vi "Sim GPS.vi"() -> ()   [LabVIEW 2012]
uses:
  <instrlib>/Garmin GPS Series/HAIOL/Simulator/Garmin GPS Series Simulator.lvclass
  <instrlib>/Garmin GPS Series/HAIOL/Garmin GPS Series.lvclass
  <vilib>/Platform/TimedLoop/XDataNode/XDataNode.xnode
  <vilib>/Platform/TimedLoop/XDataNode/nitl_modes.ctl
  <vilib>/Platform/TimedLoop/XDataNode/XDNodeRunTimeDep.lvlib
  <vilib>/Platform/TimedLoop/XDataNode/wakeup.ctl
  <vilib>/Platform/TimedLoop/XDataNode/timing_clust.ctl
panel:
  in  "error in (no error)":errorcluster
  in  "stop?":bool
  out "GPS Data":T1 {"Time"."GPS Time of Week" format="%.3f"; "Velocity, Correction & SET"."Extended Navigation Mode" items=["Non Differential"=0, "Code (RTCM Type 1 & 9)"=1, "Code, Single Frequency (WAAS)"=2, "Code, Dual Frequency (WAAS)"=3, "Code, Single Frequency (WCT)"=4, "Code/RCP, Dual Frequency (WCT)"=5, "Code, Single Frequency (RTG)"=6, "Code (RTCM Type 1 & 9) Dual Frequency"=10, "Code/RCP, Dual Frequency (RTG)"=11, "Code, Single Frequency (NCT-RTK)"=12, "Code, Single Frequency (RTCM 18 & 19)"=13, "Code, Single Frequency (RTCM 21 & 22)"=14, "Code, Single Frequency (CMR)"=15, "Code, Dual Frequency (NCT-RTK)"=16, "Code, Dual Frequency (RTCM 18 & 19)"=17, "Code, Dual Frequency (RTCM 20 & 21)"=18, "Code, Dual Frequency (CMR)"=19, "RTK (NCT-RTK)"=20, "RTK (RTCM 18 & 19)"=21, "RTK (RTCM 20 & 21)"=22, "RTK (CMR)"=23, "Code, Single Frequency with SET (RTG)"=24, "Code/RCP, Dual Frequency with SET (RTG)"=25, "RTK Extend"=26]; "Altitude" format="%#_18g"; "Longitude" format="%#_18g"; "Latitude" format="%#_18g"}
  in  "GPS Data Cluster":T1 {"Time"."GPS Time of Week" format="%.3f"; "Velocity, Correction & SET"."Extended Navigation Mode" items=["Non Differential"=0, "Code (RTCM Type 1 & 9)"=1, "Code, Single Frequency (WAAS)"=2, "Code, Dual Frequency (WAAS)"=3, "Code, Single Frequency (WCT)"=4, "Code/RCP, Dual Frequency (WCT)"=5, "Code, Single Frequency (RTG)"=6, "Code (RTCM Type 1 & 9) Dual Frequency"=10, "Code/RCP, Dual Frequency (RTG)"=11, "Code, Single Frequency (NCT-RTK)"=12, "Code, Single Frequency (RTCM 18 & 19)"=13, "Code, Single Frequency (RTCM 21 & 22)"=14, "Code, Single Frequency (CMR)"=15, "Code, Dual Frequency (NCT-RTK)"=16, "Code, Dual Frequency (RTCM 18 & 19)"=17, "Code, Dual Frequency (RTCM 20 & 21)"=18, "Code, Dual Frequency (CMR)"=19, "RTK (NCT-RTK)"=20, "RTK (RTCM 18 & 19)"=21, "RTK (RTCM 20 & 21)"=22, "RTK (CMR)"=23, "Code, Single Frequency with SET (RTG)"=24, "Code/RCP, Dual Frequency with SET (RTG)"=25, "RTK Extend"=26]}
  out "error out":errorcluster
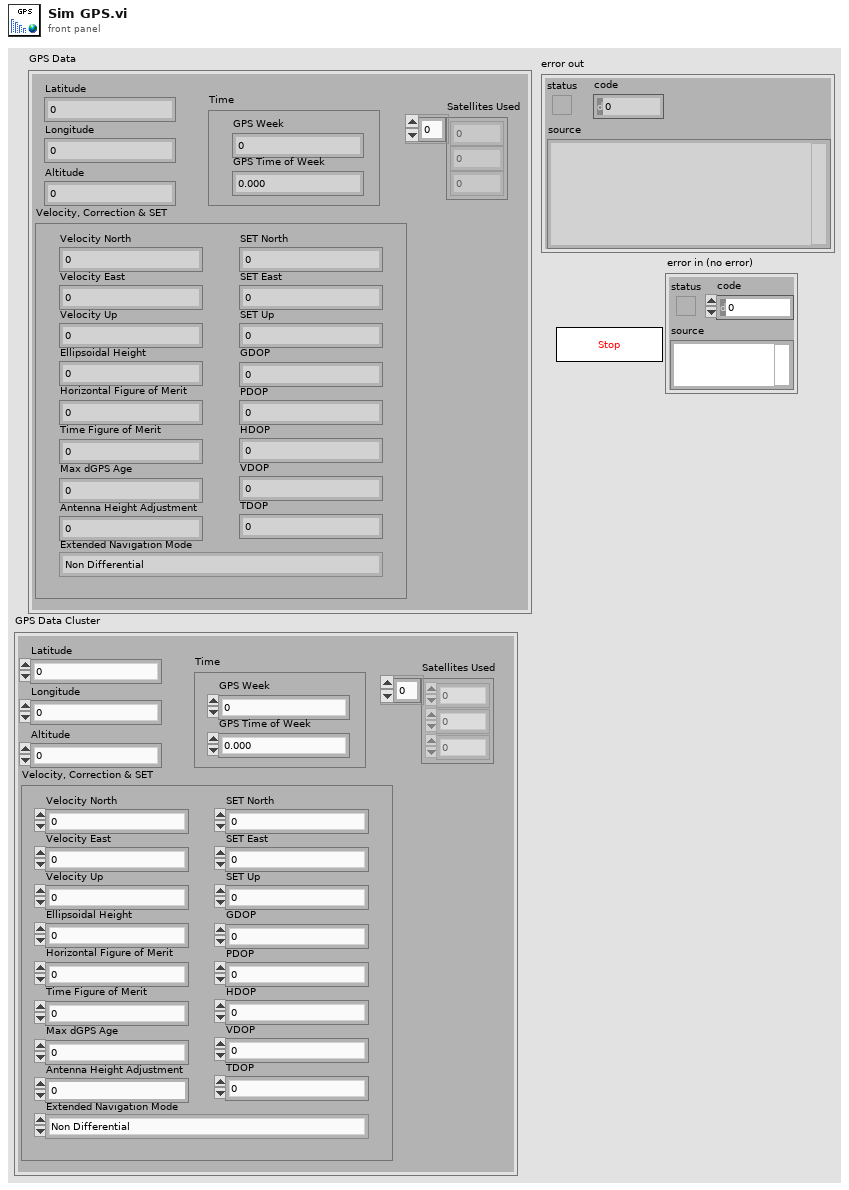
[diagram p1: front panel]
types:
  T1 = cluster{"Latitude":dbl, "Longitude":dbl, "Altitude":dbl, "Velocity, Correction & SET":cluster{"Velocity North":dbl, "Velocity East":dbl, "Velocity Up":dbl, "Ellipsoidal Height":dbl, "GDOP":sgl, "PDOP":sgl, "HDOP":sgl, "VDOP":sgl, "TDOP":sgl, "Horizontal Figure of Merit":u8, "Time Figure of Merit":u8, "Max dGPS Age":sgl, "Extended Navigation Mode":u8, "Antenna Height Adjustment ":dbl, "SET North":i32, "SET East":i32, "SET Up":i32}, "Time":cluster{"GPS Week":u16, "GPS Time of Week":sgl}, "Satellites Used":i32[]}
  T2 = typedef "XDNodeRunTimeDep.lvlib/timing_clust.ctl" = cluster{"Expected End [f-1]":u64, "Actual End [f-1]":u64, "Finished Late? [f-1]":bool, "Expected End [i-1]":u64, "Actual End [i-1]":u64, "Finished Late? [i-1]":bool, "Expected Start [i]":u64, "Actual Start [i]":u64, "Expected Start [f]":u64, "Actual Start [f]":u64, "Source Name":string, "Structure Name":string, "Period":i64, "Deadline":i64, "Offset":i64, "Start":i64, "Priority":i32, "Timeout":i32, "Mode":T3, "Wakeup Reason":T4, "Error":errorcluster, "Source Type":string, "Secondary Source Type":string, "Global End Time":u64, "Global Start Time":u64, "Frame Duration":u64, "Iteration Duration":u64, "Assigned CPU":i32, "I/O Scan Engine Mode":u32}
  T3 = typedef "XDNodeRunTimeDep.lvlib/nitl_modes.ctl" = enum32{"No Change", "Process missed periods, maintain original phase", "Discard missed periods, maintain original phase", "Process missed periods, ignore original phase", "Discard missed periods, ignore original phase"}
  T4 = typedef "XDNodeRunTimeDep.lvlib/wakeup.ctl" = enum32{"Normal", "Aborted", "Asynchronous wakeup", "Timing source error", "Timed loop error", "Timeout"}
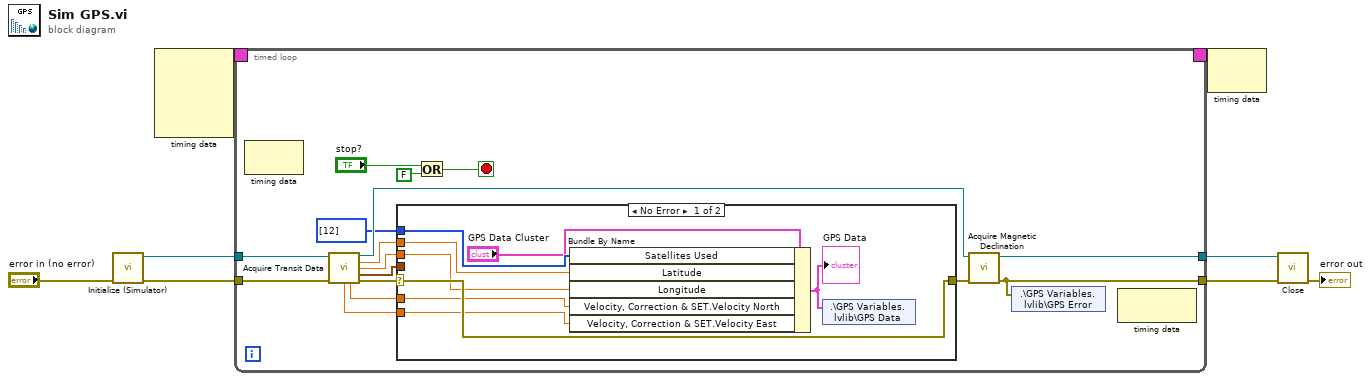
[diagram p0: block diagram]
diagram:
  n1 = call <instrlib>:"Initialize (Simulator).vi"("error in (no error)"="error in (no error)") -> ("error out"=w5:errorcluster, "Garmin GPS Series out"=w6:refnum<class "Garmin GPS Series.lvclass">)  [unwired: 9 in]
  n2 = node-c288() -> (w8:T2)  [unwired: 4 in]
  n3 = timed-loop {
    timing: w8 -> [_]
    timing-out: [_] -> w7
    tunnel: w6 -> [w24]
    tunnel: w5 -> [w23]
    tunnel: [w22] -> w4
    tunnel: [w14] -> w1
    stop <- w11 stop-if-true
    n4 = node-c288() -> ()  [unwired: 1 in, 1 out]
    n5 = call-dynamic "Acquire Transit Data.vi"("Garmin GPS Series In"=w24, "error in (no error)"=w23) -> ("Garmin GPS Series Out"=w21:refnum<class "Garmin GPS Series.lvclass">, "Latitude (degree)"=w19:dbl, "Longitude (degree)"=w18:dbl, "Time Stamp"=w20:timestamp, "Bearing (degree)"=w9:dbl, "Speed Over Ground (knots)"=w10:dbl, "error out"=w17:errorcluster)  [unwired: 7 in]
    n6 = case shown="No Error" w17 {
      selector: w17 -> [w32 w33]
      tunnel: [w32 w33] -> w16
      tunnel: w19 -> [w31 _]
      tunnel: w18 -> [w30 _]
      tunnel: i32[] [12] ("Satellites Used") -> [w29 _]
      tunnel: w20 -> [_ _]
      tunnel: w10 -> [w26 _]
      tunnel: w9 -> [w25 _]
      frame No Error {
        n7 = Bundle By Name(cluster="GPS Data Cluster", "Satellites Used"=w29, "Latitude"=w31, "Longitude"=w30, "Velocity, Correction & SET.Velocity North"=w26, "Velocity, Correction & SET.Velocity East"=w25) -> (w28:T1)
        "GPS Data" <- w28
        n8 = shared-variable ".\\GPS Variables.lvlib\\GPS Data"(w28) -> ()  [unwired: 1 in, 1 out]
      }
      frame Error {
      }
    }
    n9 = Or(x="stop?", y=FALSE) -> (x .or. y?=w11:bool)
    n10 = call-dynamic "Acquire Magnetic Declination.vi"("error in (no error)"=w16, "Garmin GPS Series In"=w21) -> ("error out"=w14:errorcluster, "Garmin GPS Series Out"=w22:refnum<class "Garmin GPS Series.lvclass">)  [unwired: 6 in, 2 out]
    n11 = shared-variable ".\\GPS Variables.lvlib\\GPS Error"(w14) -> ()  [unwired: 1 in, 1 out]
    n12 = node-c288() -> ()  [unwired: 1 in, 1 out]
  }
  n13 = node-c288(w7) -> ()  [unwired: 1 out]
  n14 = call-dynamic "Close.vi"("error in (no error)"=w1, "Garmin GPS Series in"=w4) -> ("error out"=→"error out":errorcluster)  [unwired: 9 in]
